vi "Add.vi"(10 "x":dbl, 11 "y":dbl) -> (3 "x+y":dbl)   [LabVIEW 2015]
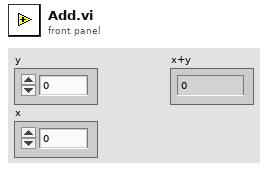
[diagram p1: front panel]
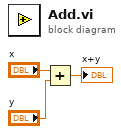
[diagram p0: block diagram]
diagram:
  n1 = Add(x="x", y="y") -> (x+y=→"x+y":dbl)
